vi "Write_I2C_Data.vi"(8 "Error_In":errorcluster, 10 "Convertor_Data":T1={"Vmin"=0.0, "Vmax"=1.0, "Input"="", "Off_Set (uS)"=0.0, "T_HD_STA (uS)"=0.0, "Sample_Per_Us"=0.0, "T_HD_DAT (uS)"=0.0, "T_SU_DAT (uS)"=0.0, "Frequency (kHz)"=0.0, "T_SU_STO"=0.0, "T_Off (uS)"=0.0, "T_On (uS)"=0.0, "T_BUF"=0.0, "Target_Address"=0, "Selected_Register_Address"=0, "Byte_Array"=[], "Target_Name"="", "Register_Name"=[], "Register_Address"=[], "Ring"=0} {"Target_Type" items=["Select Item", ""]; "Selected_Register_Address" format="%x"; "Target_Address" format="%x"}, 11 "I2C_In":refnum<class "I2C.lvclass">) -> (0 "Error_Out":errorcluster, 3 "I2C_Out":refnum<class "I2C.lvclass">)   [LabVIEW 2023, in "I2C.lvclass"]
uses:
  I2C.lvclass
  Controls/Converted_Data.ctl
  Controls/Menu_Ring.ctl
  I2C.lvclass/I2C.ctl
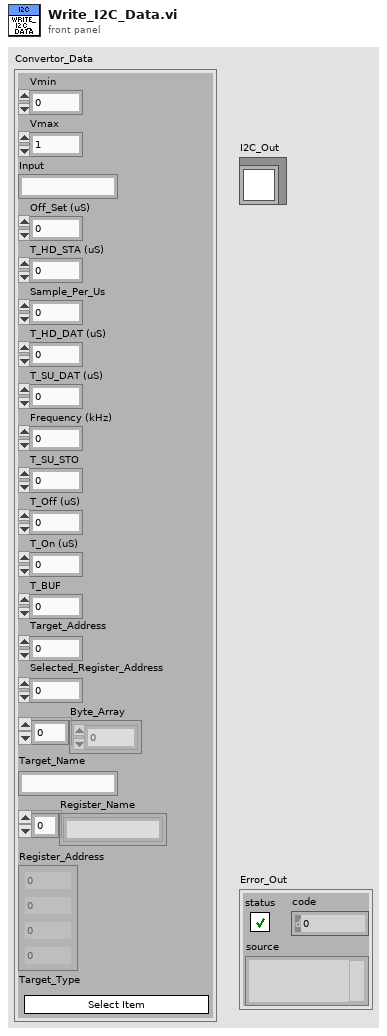
[diagram p1: front panel]
types:
  T1 = typedef "Converted_Data.ctl" = cluster{"Vmin":dbl, "Vmax":dbl, "Input":string, "Off_Set (uS)":dbl, "T_HD_STA (uS)":dbl, "Sample_Per_Us":dbl, "T_HD_DAT (uS)":dbl, "T_SU_DAT (uS)":dbl, "Frequency (kHz)":dbl, "T_SU_STO":dbl, "T_Off (uS)":dbl, "T_On (uS)":dbl, "T_BUF":dbl, "Target_Address":u16, "Selected_Register_Address":u8, "Byte_Array":u8[], "Target_Name":string, "Register_Name":string[], "Register_Address":u8[], "Ring":T2}
  T2 = typedef "Menu_Ring.ctl" = u16
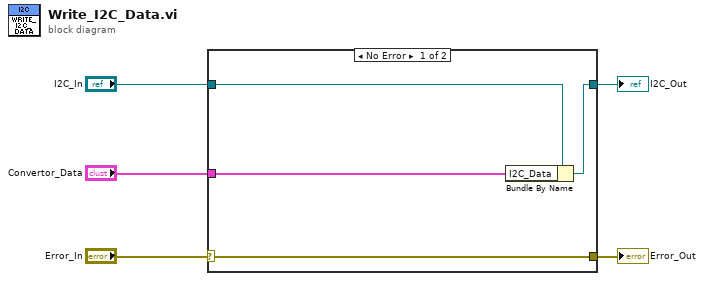
[diagram p0: block diagram]
diagram:
  n1 = case shown="No Error" "Error_In" {
    selector: "Error_In" -> [w9 w10]
    tunnel: [w9 w10] -> w4
    tunnel: [w7 w11] -> w2
    tunnel: "I2C_In" -> [w8 w11]
    tunnel: "Convertor_Data" -> [w6 _]
    frame No Error {
      n2 = Bundle By Name(cluster=w8, "I2C_Data"=w6) -> (w7:refnum<class "I2C.lvclass">)
    }
    frame Error {
    }
  }
  "Error_Out" <- w4
  "I2C_Out" <- w2
